vi "verifyQR.vi"(8 "Error In":errorcluster, 11 "Value In":string) -> (0 "Error Out":errorcluster, 2 "isValid?":bool, 3 "Value Out":string)   [LabVIEW 2018]
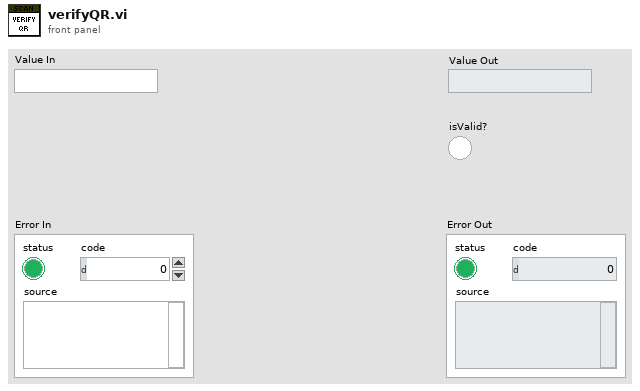
[diagram p1: front panel]
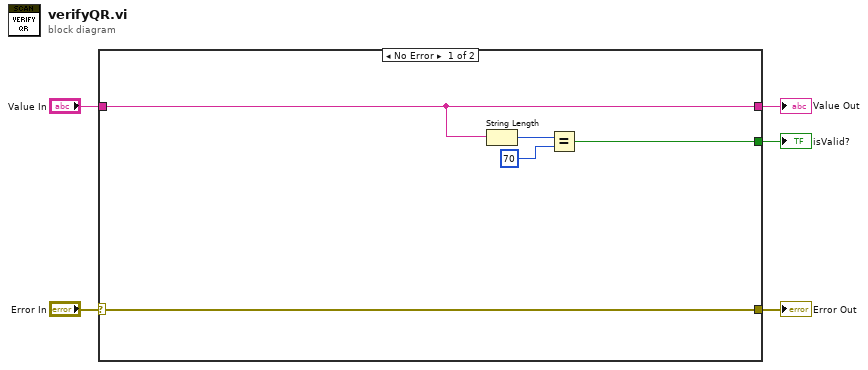
[diagram p0: block diagram]
diagram:
  n1 = case shown="No Error" "Error In" {
    selector: "Error In" -> [w10 w12]
    tunnel: [w10 w12] -> w4
    tunnel: "Value In" -> [w9 w11]
    tunnel: [w9 w11] -> w2
    tunnel: [w6 _] -> w1
    frame No Error {
      n2 = String Length(string=w9) -> (length=w8:i32)
      n3 = Equal?(x=w8, y=70) -> (x = y?=w6:bool)
    }
    frame Error {
    }
  }
  "Error Out" <- w4
  "Value Out" <- w2
  "isValid?" <- w1
